vi "Centrechamp.vi"(4 "Rot(rad)":dbl min=-120.0 max=120.0 step=1.0 format="%.5f", 5 "CentreTelY":i32=150641 max=1000000, 6 "CentreTelX":i32=29762 min=1 max=1000000, 7 "arcmin/pulse":dbl=5.367e-05 format="%.5e") -> (0 "Max Y":dbl format="%.2f", 1 "Min Y":dbl format="%.2f", 2 "Max X":dbl format="%.2f", 3 "Min X":dbl format="%.2f")   [LabVIEW 2010]
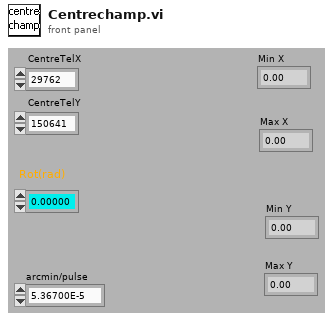
[diagram p1: front panel]
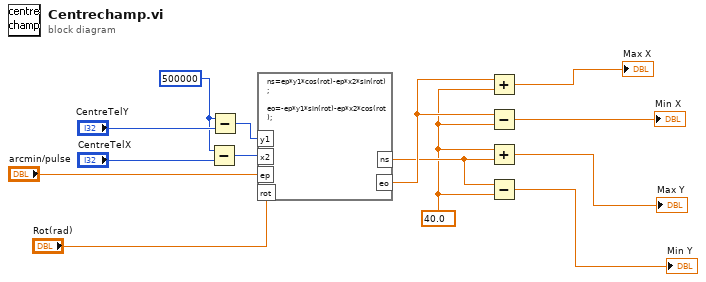
[diagram p0: block diagram]
diagram:
  w9 = 500000 ("x")
  w6 = 40.0 ("y")
  n1 = Subtract(x=w9, y="CentreTelX") -> (x-y=w14:i32)
  n2 = Subtract(x=w9, y="CentreTelY") -> (x-y=w13:i32)
  n3 = formula code="ns=ep*y1*cos(rot)-ep*x2*sin(rot);\n\neo=-ep*y1*sin(rot)-ep*x2*cos(rot);"("y1"=w13, "x2"=w14, "ep"="arcmin/pulse", "rot"="Rot(rad)") -> ("eo"=w12:dbl, "ns"=w7:dbl)
  n4 = Add(x=w12, y=w6) -> (x+y=→"Max X":dbl)
  n5 = Subtract(x=w12, y=w6) -> (x-y=→"Min X":dbl)
  n6 = Add(x=w6, y=w7) -> (x+y=→"Max Y":dbl)
  n7 = Subtract(x=w7, y=w6) -> (x-y=→"Min Y":dbl)
